vi "Read Waveform Measurement [WM] Core.vi"(0 "CS++Scope":refnum<class "CS++Scope.lvclass">, 5 "channel name (\"CHANNEL1\")":string="CHANNEL1", 7 "measurement function (Rise Time)":i32(ring) items=["Rise Time"=0, "Fall Time"=1, "Frequency"=2, "Period"=3, "Voltage RMS"=4, "Voltage RMS (cycle)"=16, "Voltage Min"=7, "Voltage Max"=6, "Voltage Vpp"=5, "Voltage Low"=9, "Voltage High"=8, "Voltage Average"=10, "Voltage Average (cycle)"=17, "Width Negative"=11, "Width Positive"=12, "Duty Cycle Negative"=13, "Duty Cycle Positive"=14, "Amplitude"=15, "Overshoot"=18, "Preshoot"=19], 9 "maximum time (5000ms)":i32=5000, 11 "error in (no error)":errorcluster) -> (4 "CS++Scope out":refnum<class "CS++Scope.lvclass">, 6 "measurement":dbl format="%^.2e", 15 "error out":errorcluster)   [LabVIEW 2013, in "CS++Scope.lvlib" / "CS++Scope.lvclass"]
doc: "This VI initiates an acquisition on all channels that you enable with the IviScope Configure Channel VI. If the channel you specify in the Channel Name parameter is not enabled for the acquisition, this VI returns the IVISCOPE_ERROR_CHANNEL_NOT_ENABLED (0xBFFA2001) error. It then waits for the acquisition to complete and returns the waveform measurement for the channel you specify. If the oscilloscope did not complete the acquisition within the time period you specify with the Maximum Time parameter, the VI returns the IVISCOPE_ERROR_MAX_TIME_EXCEEDED (0xBFFA2003) error.\n\nYou call the IviScope Fetch Waveform Measurement [WM] VI to obtain any other waveform measurement on a specific channel without initiating another acquisition.\n\nNotes:\n(1) You must configure the appropriate reference levels before you call this VI. You configure the low, mid, and high references either by calling the IviScope Configure Reference Levels [WM] VI or by setting the following properties:\nIviScope>>Waveform Measurement [WM]>> Measurement High Reference [WM]\nIviScope>>Waveform Measurement [WM]>> Measurement Low Reference [WM]\nIviScope>>Waveform Measurement [WM]>> Measurement Mid Reference [WM]\n\n(2) This VI performs interchangeability checking when the IviScope>>Inherent IVI Settings>>User Options>>Interchange Check property is set to TRUE. If the IviScope>>Inherent IVI Settings>>User Options>>Spy property is set to TRUE, you use the NI I/O Trace utility to view interchangeability warnings. You use the IviScope Get Next Interchange Warning VI to retrieve interchangeability warnings when the IviScope>>Inherent IVI Settings>>User Options>>Spy property is set to FALSE. For more information about interchangeability checking, refer to the help text for the IviScope>>Inherent IVI Settings>>User Options>>Interchange Check property.\n\n(3) The class driver returns a simulated measurement when this VI is called and the IviScope>>Inherent IVI Settings>>User Options>>Simulate property is set to TRUE and the IviScope>>Inherent IVI Settings>>User Options>>Use Specific Simulation property is set to FALSE. For information on how to configure a simulated measurement, refer to the online help manual.\n\n(4) This VI is part of the IviScopeWaveformMeasurement [WM] extension group."
uses:
  CS++Scope.lvclass
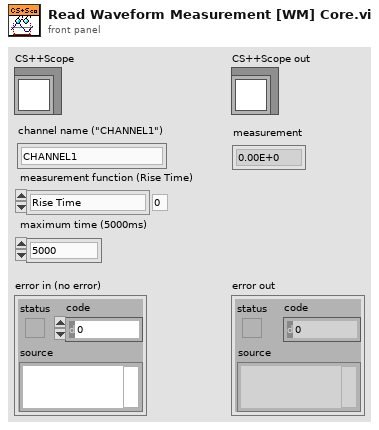
[diagram p1: front panel]
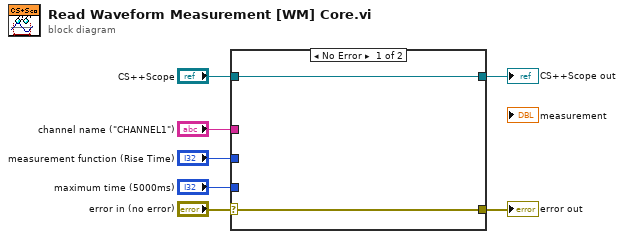
[diagram p0: block diagram]
diagram:
  n1 = case shown="No Error" "error in (no error)" {
    selector: "error in (no error)" -> [w8 w11]
    tunnel: [w8 w11] -> w6
    tunnel: [w9 w10] -> w2
    tunnel: "CS++Scope" -> [w9 w10]
    tunnel: "channel name (\"CHANNEL1\")" -> [_ _]
    tunnel: "measurement function (Rise Time)" -> [_ _]
    tunnel: "maximum time (5000ms)" -> [_ _]
    frame No Error {
    }
    frame Error {
    }
  }
  "error out" <- w6
  "CS++Scope out" <- w2
